vi "Autonomous Independent.vi"() -> ()   [LabVIEW 2012]
doc: "This VI is called when autonomous begins, and will automatically be terminated when autonomous ends. You can carry out timed or sensor driven robot movement independently without needing to return to the caller."
uses:
  <vilib>/Rock Robotics/WPI/Solenoid/WPI_SolenoidValue.ctl
  Robot Global Data.vi
  <vilib>/Rock Robotics/WPI/Joystick/WPI_JoystickGetSetRefNum.vi
  <vilib>/Rock Robotics/WPI/Solenoid/WPI_SolenoidSetEnum.vi
  <vilib>/addons/control/pid/pid.llb/PID (DBL).vi
  <vilib>/addons/control/pid/NI_PID_pid.lvlib
panel:
  in  "StraightPID gains 2":T1={"proportional gain (Kc)"=0.2, "integral time (Ti, min)"=0.0, "derivative time (Td, min)"=0.0} {"derivative time (Td, min)" format="%.3f"; "integral time (Ti, min)" format="%.3f"; "proportional gain (Kc)" format="%.3f"}
  in  "distance to bridge":dbl=4.1
  in  "Min Speed Bridge":dbl=0.1
  out "Distance Shoot":dbl[](array[numeric])=[0.5463065049614113, 0.4884233737596472] format="%#_4f"
  out "Distance Bridge":dbl[](array[numeric])=[15.640573318632855, 16.066427783902977] format="%#_4f"
  in  "Bridge approach\nSpeed":dbl=0.25
  in  "StraightPID gains":T1={"proportional gain (Kc)"=0.2, "integral time (Ti, min)"=0.0, "derivative time (Td, min)"=0.0} {"derivative time (Td, min)" format="%.3f"; "integral time (Ti, min)" format="%.3f"; "proportional gain (Kc)" format="%.3f"}
  in  "Shooter approach\nSpeed":dbl=-0.25
  out "Header":dbl
  in  "Min Speed Shoot":dbl=-0.1
  in  "Enum":enum16{"Straight", "Right", "Left", "Vision"}(ring)
  in  "PID gains":T1={"proportional gain (Kc)"=0.1, "integral time (Ti, min)"=0.0, "derivative time (Td, min)"=0.0} {"derivative time (Td, min)" format="%.3f"; "integral time (Ti, min)" format="%.3f"; "proportional gain (Kc)" format="%.3f"}
  out "Heading":dbl
  in  "Min Distance (ft)":dbl=3.25
  in  "inRange Power":dbl=-0.3
  out "Distance (ft)":dbl
  in  "inRange distance (ft)":dbl=4.0
  in  "Reverse Power":dbl=0.2
  in  "Camera Position":T2={"Radius (in)"=0.0, "Height (in)"=39.0, "Vertical Angle"=0.0}
  # "This assumes that the camera\nis facing directly out from the \ncenter of the robot"
  # "Distance from camera to \naxis of rotation on the robot"
  # "Example:"
  # "-0.1"
  # "4"
  # "0.1"
  # "-.25"
  # ".200"
  # ".25"
  # "Axis of rotation"
  # "Camera"
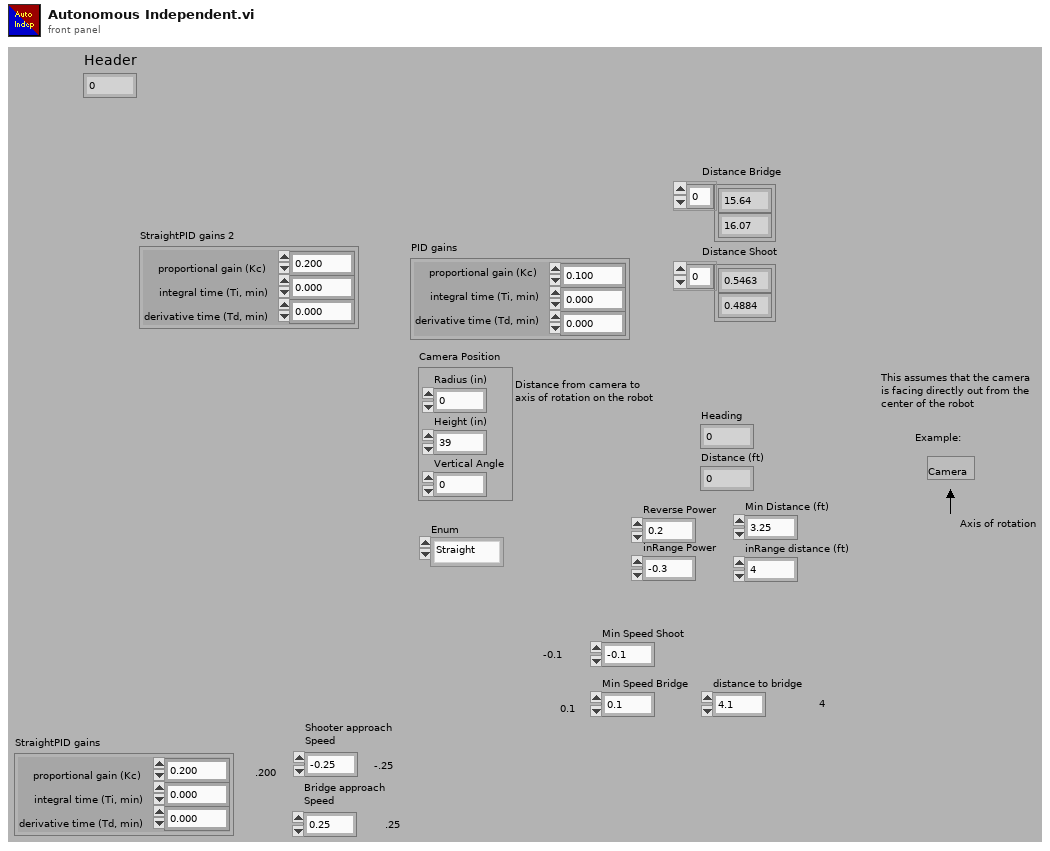
[diagram p1: front panel]
types:
  T1 = cluster{"proportional gain (Kc)":dbl, "integral time (Ti, min)":dbl, "derivative time (Td, min)":dbl}
  T2 = cluster{"Radius (in)":dbl, "Height (in)":dbl, "Vertical Angle":dbl}
  T3 = typedef "WPI_JoystickDevRef.ctl" = cluster{"Device":T4}
  T4 = typedef "WPI_JoystickDeviceEnum.ctl" = enum16{"USB 1", "USB 2", "USB 3", "USB 4", "Kinect 1", "Kinect 2"}
  T5 = cluster{"axis 1 (x)":dbl, "axis 2 (y)":dbl, "axis 3 (throttle)":dbl, "axis 4":dbl, "axis 5":dbl, "axis 6":dbl}
  T6 = typedef "WPI_MotorControlDeviceRef.ctl" = cluster{"DeviceStatus":errorcluster, "Type":enum16{"PWM", "CAN"}, "PWM":cluster{"Digital Module":T7, "PWM Channel":T8, "DeadBand":T9}, "CAN":cluster{"Device Number":u8, "Control Mode":T10, "Semaphore":T11, "Max Vout":dbl}, "Invert":bool, "TransformRef":T12, "InvTransformRef":T12}
  T7 = typedef "FPGA_TypedefDigitalModule.ctl" = enum16{"Digital Module 1", "Digital Module 2"}
  T8 = typedef "FPGA_DIOPWMChannel.ctl" = enum8{"PWM 1", "PWM 2", "PWM 3", "PWM 4", "PWM 5", "PWM 6", "PWM 7", "PWM 8", "PWM 9", "PWM 10", "Invalid"}
  T9 = typedef "WPI_PWMDeadband.ctl" = cluster{"Name":string, "maxPositivePwm":i32, "minPositivePwm":i32, "centerPwm":i32, "maxNegativePwm":i32, "minNegativePwm":i32, "angularRange":u16}
  T10 = typedef "WPI_CANJaguar_ControlMode.ctl" = enum8{"Percent VBus", "Current", "Speed", "Position", "Voltage"}
  T11 = typedef "Semaphore RefNum" = refnum<k1>
  T12 = typedef "WPI_PWMTransform_ConPane.ctl" = refnum<vi>
  T13 = typedef "WPI_SolenoidValue.ctl" = enum16{"Off", "On", "Forward", "Reverse"}
  T14 = typedef "WPI_SolenoidDevRef.ctl" = cluster{"DevStatus":errorcluster, "Solenoid Module":T15, "Forward Solenoid Channel":T16, "Reverse Solenoid Channel":T16}
  T15 = typedef "FPGA_TypedefSolenoidModule.ctl" = enum16{"Solenoid Module 1", "Solenoid Module 2"}
  T16 = typedef "WPI_SolenoidChannel.ctl" = enum8{"Solenoid 1", "Solenoid 2", "Solenoid 3", "Solenoid 4", "Solenoid 5", "Solenoid 6", "Solenoid 7", "Solenoid 8", "Invalid"}
  T17 = cluster{"Position":cluster{"X":dbl, "Y":dbl}, "Distance (ft)":dbl, "Angle Offset":dbl, "Bounding Box":cluster{"Left":dbl, "Top":dbl, "Right":dbl, "Bottom":dbl}}[]
  T18 = cluster{"Position":cluster{"X":dbl, "Y":dbl}, "Distance (ft)":dbl, "Angle Offset":dbl, "Bounding Box":cluster{"Left":dbl, "Top":dbl, "Right":dbl, "Bottom":dbl}}
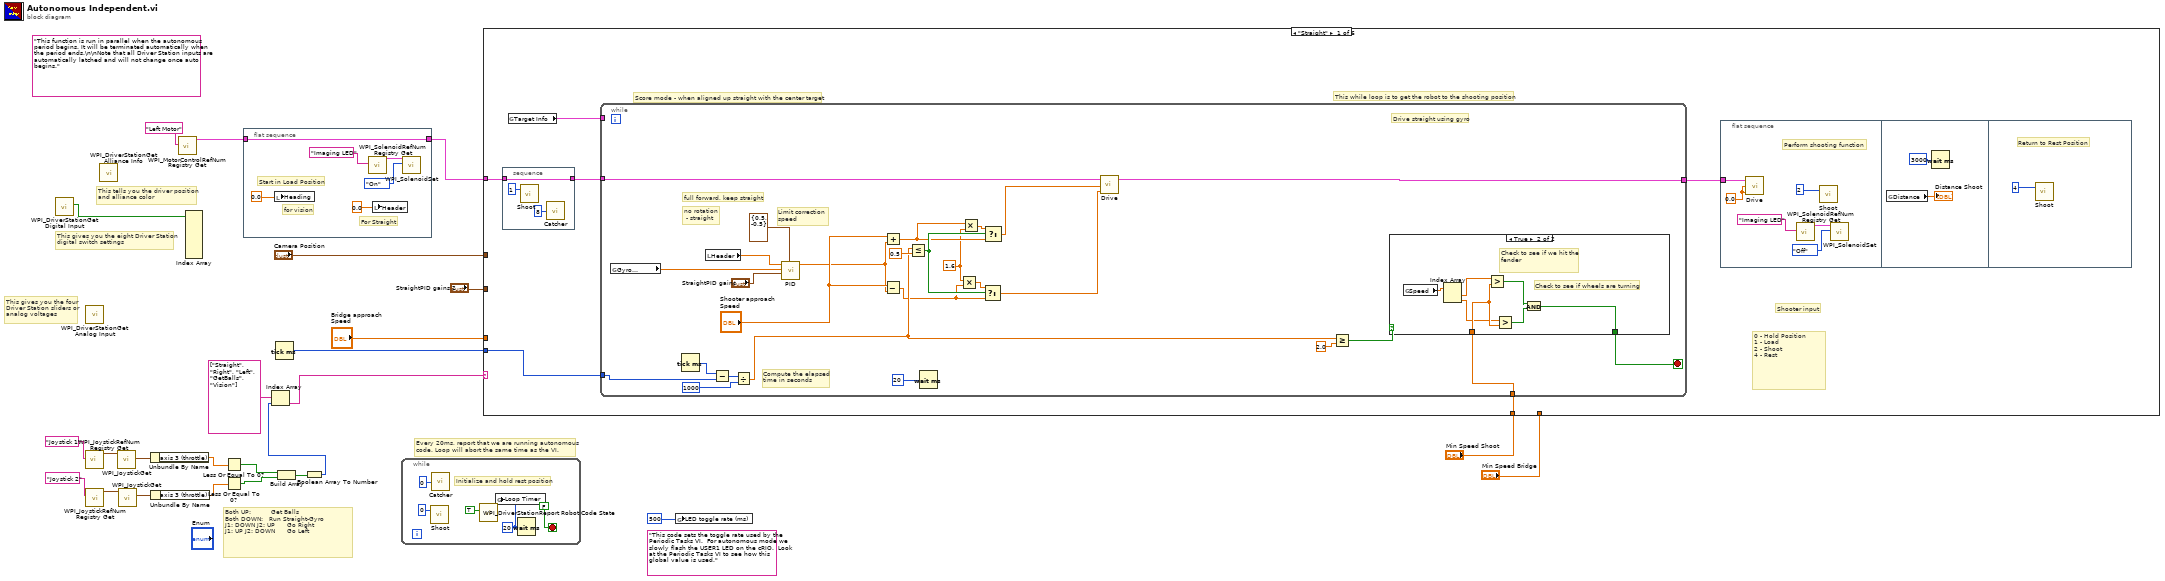
[diagram p0: block diagram]
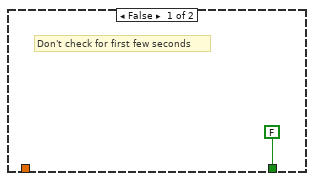
[diagram p2: hidden frame]
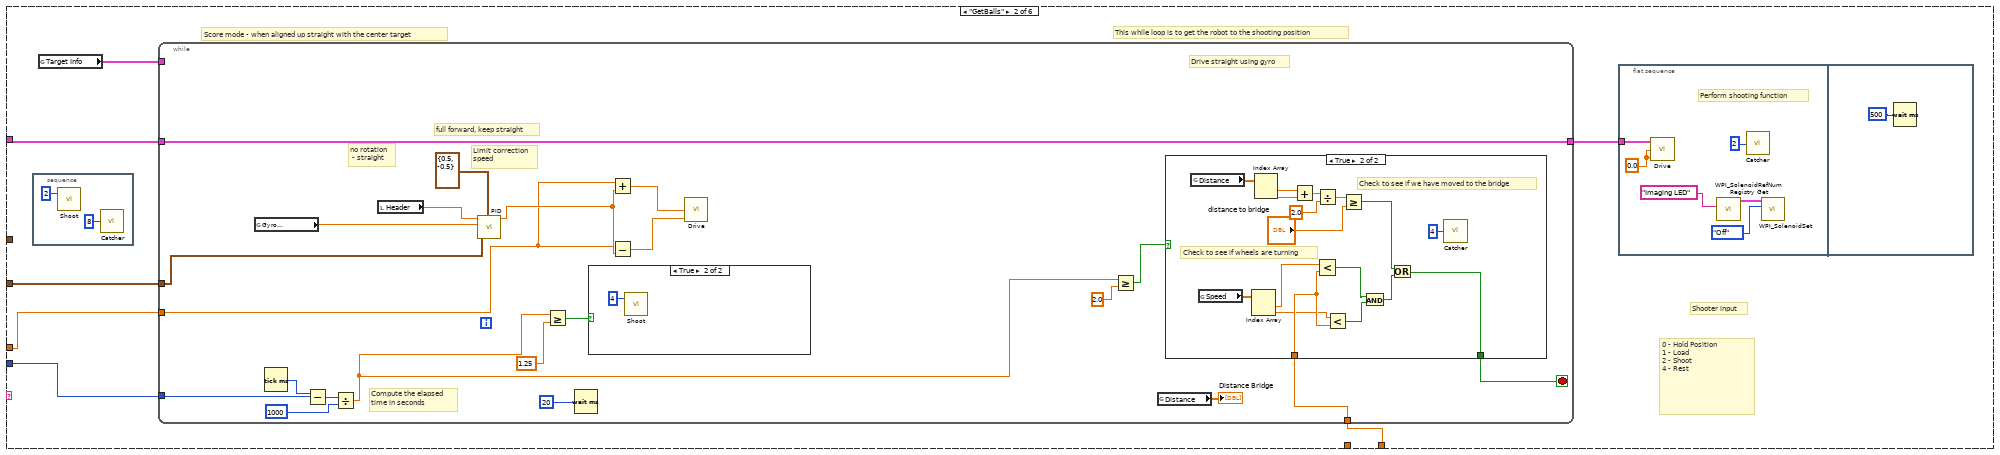
[diagram p3: hidden frame]
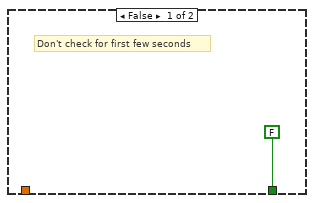
[diagram p5: hidden frame]
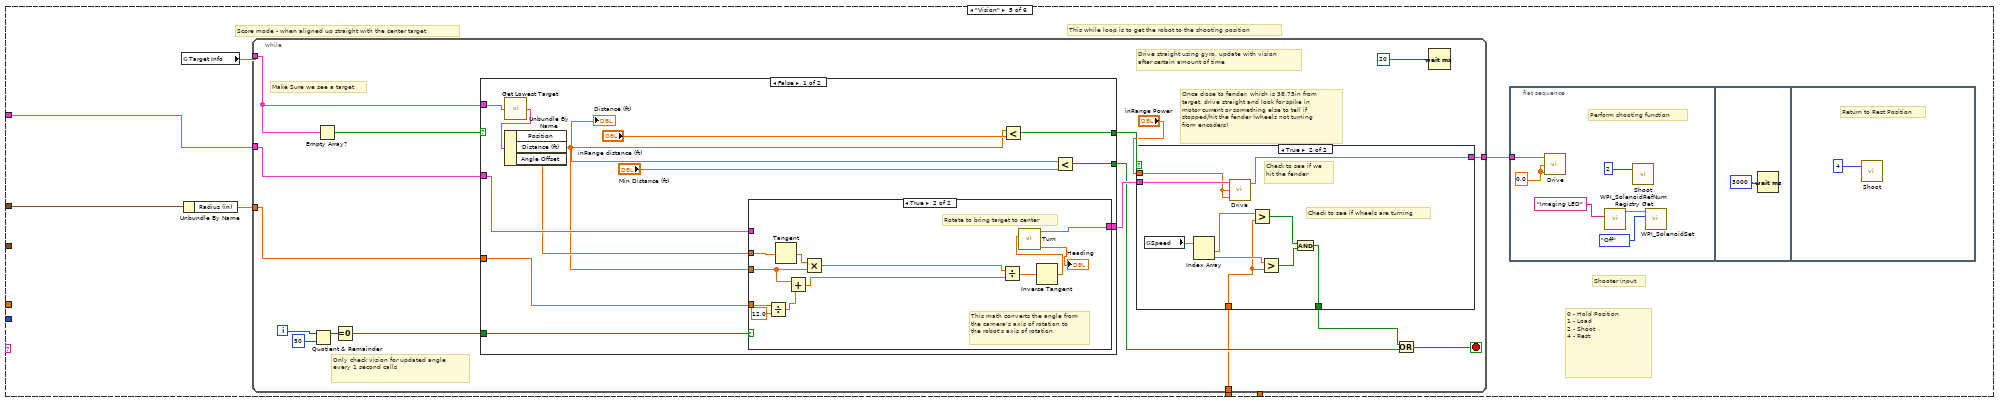
[diagram p8: hidden frame]
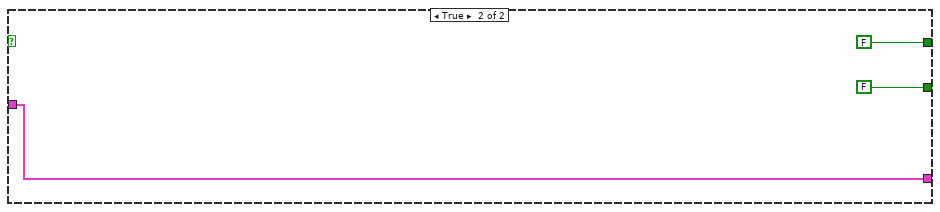
[diagram p10: hidden frame]
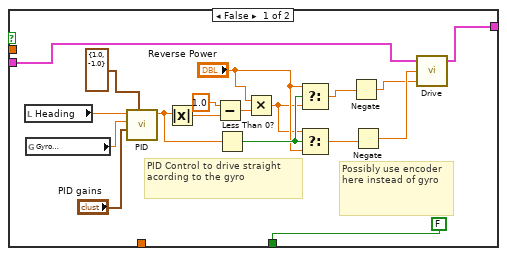
[diagram p11: hidden frame]
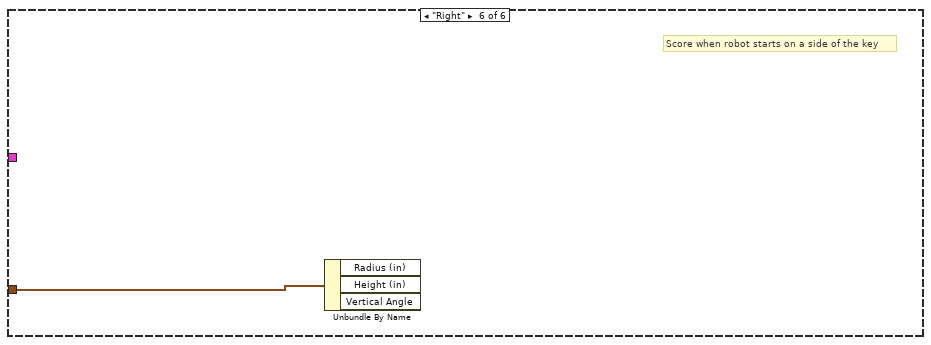
[diagram p12: hidden frame]
diagram:
  (unwired) "This code sets the toggle rate used by the Periodic Tasks VI.  For autonomous mode we slowly flash the USER1 LED on the cRIO.  Look at the Periodic Tasks VI to see how this global value is used."
  (unwired) "This function is run in parallel when the autonomous period begins. It will be terminated automatically when the period ends.\n\nNote that all Driver Station inputs are automatically latched and will not change once auto begins."
  # "Both UP:          Get Balls\nBoth DOWN:   Run Straight-Gyro\nJ1: DOWN J2: UP      Go Right\nJ1: UP J2: DOWN      Go Left"
  # "Every 20ms, report that we are running autonomous\ncode. Loop will abort the same time as the VI."
  # "This tells you the driver position\nand alliance color"
  # "This gives you the eight Driver Station\ndigital switch settings"
  # "This gives you the four\nDriver Station sliders or\nanalog voltages"
  n1 = call <vilib>:"WPI_DriverStationGet Digital Input.vi"() -> ("Driver Station Digital Input (1-8)"=w25:bool[])  [unwired: 11 out]
  n2 = call <vilib>:"WPI_JoystickRefNum Registry Get.vi"("refnum name"="Joystick 1") -> ("JoystickDevRef"=w14:T3)  [unwired: 1 in, 9 out]
  n3 = call <vilib>:"WPI_DriverStationGet Analog Input.vi"() -> ()  [unwired: 12 out]
  n4 = call <vilib>:"WPI_JoystickRefNum Registry Get.vi"("refnum name"="Joystick 2") -> ("JoystickDevRef"=w11:T3)  [unwired: 1 in, 9 out]
  n5 = call <vilib>:"WPI_DriverStationGet Alliance Info.vi"() -> ()  [unwired: 12 out]
  n6 = call <vilib>:"WPI_JoystickGet.vi"("JoystickDevRef"=w14) -> ("Axes"=w15:T5)  [unwired: 1 in, 5 out]
  n7 = call <vilib>:"WPI_JoystickGet.vi"("JoystickDevRef"=w11) -> ("Axes"=w10:T5)  [unwired: 1 in, 5 out]
  n8 = Unbundle By Name(w15) -> ("axis 3 (throttle)"=w13:dbl)
  n9 = Unbundle By Name(w10) -> ("axis 3 (throttle)"=w12:dbl)
  n10 = call <vilib>:"WPI_MotorControlRefNum Registry Get.vi"("refnum name"="Left Motor") -> ("MotorControlDevRef"=w5:T6)  [unwired: 9 in, 1 out]
  n11 = Index Array(array=w25) -> ()  [unwired: 8 in, 8 out]
  n12 = Less Or Equal To 0?(x=w13) -> (x <= 0?=w6:bool)
  n13 = Less Or Equal To 0?(x=w12) -> (x <= 0?=w7:bool)
  n14 = flat-sequence {
    tunnel: [w31] -> w4
    tunnel: w5 -> [w31]
    frame #0 {
      # "For Straight"
      # "for vision"
      # "Start in Load Position"
      n15 = local write "Heading"(0.0 ("Heading")) -> ()
      n16 = call <vilib>:"WPI_SolenoidRefNum Registry Get.vi"("refnum name"="Imaging LED") -> ("SolenoidDevRef"=w29:T14)  [unwired: 9 in, 1 out]
      n17 = local write "Header"(0.0 ("Header")) -> ()
      n18 = call-poly <vilib>:"WPI_SolenoidSet.vi"("Value"=WPI_SolenoidValue."On", "SolenoidDevRef"=w29) -> ()  [unwired: 8 in, 2 out]
    }
  }
  n19 = Tick Count (ms)() -> (millisecond timer value=w18:u32)
  n20 = Build Array(w6, w7) -> (w8:bool[])
  n21 = Boolean Array To Number(Boolean array=w8) -> (number=w22:u32)
  n22 = Index Array(array=string[] ["Straight", "Right", "Left", "GetBalls", "Vision"], index=w22) -> (element=w21:string)
  n23 = while {
    stop <- FALSE stop-if-true
    w33 = u32 20 ("milliseconds to wait")
    # "Initialize and hold rest position"
    n24 = call "Shoot.vi"("Shooter Position (0 to 8)"=i8 0 ("Shooter Position (0 to 4)")) -> ()  [unwired: 1 in, 2 out]
    n25 = call "Catcher.vi"("Catcher Position"=i8 0) -> ()
    n26 = call <vilib>:"WPI_DriverStationReport Robot Code State.vi"("Autonomous"=TRUE) -> ()  [unwired: 10 in, 1 out]
    n27 = global write "Robot Global Data.vi" "Loop Timer"(w33) -> ()
    n28 = Wait (ms)(milliseconds to wait=w33) -> ()  [unwired: 1 out]
  }
  n29 = case shown="\"Straight\"" w21 {
    tunnel: w4 -> [w38 w94 _ _ w151 _]
    tunnel: "Camera Position" -> [_ _ _ _ w150 w234]
    tunnel: w18 -> [w40 w93 _ _ _ _]
    tunnel: "Min Speed Shoot" -> [w39 _ _ _ w147 _]
    tunnel: "Bridge approach\nSpeed" -> [_ w92 _ _ _ _]
    tunnel: "Min Speed Bridge" -> [_ w91 _ _ _ _]
    tunnel: "StraightPID gains 2" -> [_ w90 _ _ _ _]
    frame "Straight" {
      # "Shooter input"
      # "0 - Hold Position\n1 - Load\n2 - Shoot\n4 - Rest"
      # "This while loop is to get the robot to the shooting position"
      # "Score mode - when aligned up straight with the center target"
      n30 = stacked-sequence {
        tunnel: [w43] -> w37
        tunnel: w38 -> [w43]
        frame #0 {
          n31 = call "Shoot.vi"("Shooter Position (0 to 8)"=i8 1 ("Shooter Position (0 to 4)")) -> ()  [unwired: 1 in, 2 out]
          n32 = call "Catcher.vi"("Catcher Position"=i8 8) -> ()
        }
      }
      n33 = global read "Robot Global Data.vi" "Target Info"() -> (w42:T17)
      n34 = while {
        tunnel: w42 -> [_]
        tunnel: w37 -> [w70]
        tunnel: [w69] -> w41
        tunnel: w40 -> [w77]
        tunnel: w39 -> [w76]
        stop <- w75 stop-if-true
        w56 = 1.6 ("y")
        # "full forward, keep straight"
        # "Limit correction\nspeed"
        # "no rotation\n - straight"
        # "Compute the elapsed\ntime in seconds"
        # "Drive straight using gyro"
        n35 = global read "Robot Global Data.vi" "Gyro\nAngle"() -> (w67:dbl)
        n36 = Tick Count (ms)() -> (millisecond timer value=w80:u32)
        n37 = local read "Header"() -> (w65:dbl)
        n38 = Subtract(x=w80, y=w77) -> (x-y=w78:u32)
        n39 = Divide(x=w78, y=u32 1000 ("milliseconds to wait")) -> (x/y=w71:dbl)
        n40 = call-poly <vilib>:"PID.vi"("output range"=cluster{"output high":dbl, "output low":dbl} {"output high"=0.5, "output low"=-0.5}, "PID gains"="StraightPID gains", "process variable"=w67, "setpoint"=w65) -> ("output"=w62:dbl)  [unwired: 2 in, 5 out]
        n41 = Subtract(x="Shooter approach\nSpeed", y=w62) -> (x-y=w55:dbl)
        n42 = Add(x="Shooter approach\nSpeed", y=w62) -> (x+y=w58:dbl)
        n43 = Less Or Equal?(x=w71, y=0.5) -> (x <= y?=w63:bool)
        n44 = Wait (ms)(milliseconds to wait=u32 20) -> ()  [unwired: 1 out]
        n45 = Multiply(x=w56, y=w55) -> (x*y=w57:dbl)
        n46 = Multiply(x=w58, y=w56) -> (x*y=w59:dbl)
        n47 = Select(t=w57, s=w63, f=w55) -> (s? t:f=w60:dbl)
        n48 = Select(t=w59, s=w63, f=w58) -> (s? t:f=w61:dbl)
        n49 = call "Drive.vi"("Right Motor IN"=w60, "Left Motor IN"=w61, "Motor DevRef"=w70) -> ("Motor DevRef"=w69:T6)  [unwired: 2 in]
        n50 = Greater Or Equal?(x=w71, y=2.0) -> (x >= y?=w74:bool)
        n51 = case shown="True" w74 {
          tunnel: w76 -> [_ w89]
          tunnel: [FALSE w88] -> w75
          frame False {
            # "Don't check for first few seconds"
          }
          frame True {
            # "Check to see if wheels are turning"
            # "Check to see if we hit the fender"
            n52 = global read "Robot Global Data.vi" "Speed"() -> (w85:dbl[])
            n53 = Index Array(array=w85) -> (element #1=w84:dbl, element #2=w83:dbl)  [unwired: 2 in]
            n54 = Greater?(x=w84, y=w89) -> (0:w87:bool)
            n55 = Greater?(x=w83, y=w89) -> (0:w86:bool)
            n56 = And(x=w87, y=w86) -> (x .and. y?=w88:bool)
          }
        }
      }
      n57 = flat-sequence {
        tunnel: w41 -> [w50]
        frame #0 {
          w51 = 0.0 ("RightSpeed")
          # "Perform shooting function"
          n58 = call "Drive.vi"("Right Motor IN"=w51, "Left Motor IN"=w51, "Motor DevRef"=w50) -> ()  [unwired: 2 in, 1 out]
          n59 = call <vilib>:"WPI_SolenoidRefNum Registry Get.vi"("refnum name"="Imaging LED") -> ("SolenoidDevRef"=w48:T14)  [unwired: 9 in, 1 out]
          n60 = call "Shoot.vi"("Shooter Position (0 to 8)"=i8 2 ("Shooter Position (0 to 3)")) -> ()  [unwired: 1 in, 2 out]
          n61 = call-poly <vilib>:"WPI_SolenoidSet.vi"("Value"=WPI_SolenoidValue."Off", "SolenoidDevRef"=w48) -> ()  [unwired: 8 in, 2 out]
        }
        frame #1 {
          n62 = global read "Robot Global Data.vi" "Distance"() -> (→"Distance Shoot":dbl[])
          n63 = Wait (ms)(milliseconds to wait=u32 3000) -> ()  [unwired: 1 out]
        }
        frame #2 {
          # "Return to Rest Position"
          n64 = call "Shoot.vi"("Shooter Position (0 to 8)"=i8 4 ("Shooter Position (0 to 3)")) -> ()  [unwired: 1 in, 2 out]
        }
      }
    }
    frame "GetBalls" {
      # "Shooter input"
      # "0 - Hold Position\n1 - Load\n2 - Shoot\n4 - Rest"
      # "This while loop is to get the robot to the shooting position"
      # "Score mode - when aligned up straight with the center target"
      n65 = stacked-sequence {
        frame #0 {
          n66 = call "Shoot.vi"("Shooter Position (0 to 8)"=i8 2 ("Shooter Position (0 to 4)")) -> ()  [unwired: 1 in, 2 out]
          n67 = call "Catcher.vi"("Catcher Position"=i8 8) -> ()
        }
      }
      n68 = global read "Robot Global Data.vi" "Target Info"() -> (w96:T17)
      n69 = while {
        tunnel: w96 -> [_]
        tunnel: w94 -> [w121]
        tunnel: [w121] -> w95
        tunnel: w93 -> [w123]
        tunnel: w91 -> [w122]
        tunnel: w92 -> [w111]
        tunnel: w90 -> [w110]
        stop <- w120 stop-if-true
        # "Limit correction\nspeed"
        # "no rotation\n - straight"
        # "full forward, keep straight"
        # "Compute the elapsed\ntime in seconds"
        # "Drive straight using gyro"
        n70 = global read "Robot Global Data.vi" "Gyro\nAngle"() -> (w119:dbl)
        n71 = Tick Count (ms)() -> (millisecond timer value=w126:u32)
        n72 = Subtract(x=w126, y=w123) -> (x-y=w124:u32)
        n73 = Divide(x=w124, y=u32 1000 ("milliseconds to wait")) -> (x/y=w107:dbl)
        n74 = local read "Header"() -> (w117:dbl)
        n75 = call-poly <vilib>:"PID.vi"("output range"=cluster{"output high":dbl, "output low":dbl} {"output high"=0.5, "output low"=-0.5}, "PID gains"=w110, "process variable"=w119, "setpoint"=w117) -> ("output"=w116:dbl)  [unwired: 2 in, 5 out]
        n76 = Greater Or Equal?(x=w107, y=1.25) -> (x >= y?=w106:bool)
        n77 = Wait (ms)(milliseconds to wait=u32 20) -> ()  [unwired: 1 out]
        n78 = case shown="True" w106 {
          frame False {
          }
          frame True {
            n79 = call "Shoot.vi"("Shooter Position (0 to 8)"=i8 4 ("Shooter Position (0 to 4)")) -> ()  [unwired: 1 in, 2 out]
          }
        }
        n80 = Subtract(x=w111, y=w116) -> (x-y=w114:dbl)
        n81 = Add(x=w111, y=w116) -> (x+y=w115:dbl)
        n82 = call "Drive.vi"("Right Motor IN"=w114, "Left Motor IN"=w115) -> ()  [unwired: 3 in, 1 out]
        n83 = Greater Or Equal?(x=w107, y=2.0) -> (x >= y?=w113:bool)
        n84 = global read "Robot Global Data.vi" "Distance"() -> (→"Distance Bridge":dbl[])
        n85 = case shown="True" w113 {
          tunnel: w122 -> [_ w146]
          tunnel: [FALSE w131] -> w120
          frame False {
            # "Don't check for first few seconds"
          }
          frame True {
            # "Check to see if we have moved to the bridge"
            # "Check to see if wheels are turning"
            n86 = global read "Robot Global Data.vi" "Distance"() -> (w140:dbl[])
            n87 = global read "Robot Global Data.vi" "Speed"() -> (w143:dbl[])
            n88 = Index Array(array=w143) -> (element #1=w142:dbl, element #2=w141:dbl)  [unwired: 2 in]
            n89 = Index Array(array=w140) -> (element #1=w139:dbl, element #2=w138:dbl)  [unwired: 2 in]
            n90 = Add(x=w139, y=w138) -> (x+y=w137:dbl)
            n91 = Less?(x=w142, y=w146) -> (x < y?=w145:bool)
            n92 = Divide(x=w137, y=2.0) -> (x/y=w135:dbl)
            n93 = Less?(x=w141, y=w146) -> (x < y?=w144:bool)
            n94 = Greater Or Equal?(x=w135, y="distance to bridge") -> (x >= y?=w132:bool)
            n95 = And(x=w145, y=w144) -> (x .and. y?=w133:bool)
            n96 = Or(x=w132, y=w133) -> (x .or. y?=w131:bool)
            n97 = call "Catcher.vi"("Catcher Position"=i8 4) -> ()
          }
        }
      }
      n98 = flat-sequence {
        tunnel: w95 -> [w103]
        frame #0 {
          w104 = 0.0 ("RightSpeed")
          # "Perform shooting function"
          n99 = call "Drive.vi"("Right Motor IN"=w104, "Left Motor IN"=w104, "Motor DevRef"=w103) -> ()  [unwired: 2 in, 1 out]
          n100 = call <vilib>:"WPI_SolenoidRefNum Registry Get.vi"("refnum name"="Imaging LED") -> ("SolenoidDevRef"=w102:T14)  [unwired: 9 in, 1 out]
          n101 = call "Catcher.vi"("Catcher Position"=i8 2) -> ()
          n102 = call-poly <vilib>:"WPI_SolenoidSet.vi"("Value"=WPI_SolenoidValue."Off", "SolenoidDevRef"=w102) -> ()  [unwired: 8 in, 2 out]
        }
        frame #1 {
          n103 = Wait (ms)(milliseconds to wait=u32 500) -> ()  [unwired: 1 out]
        }
      }
    }
    frame Default {
      # "Default, Do nothing"
    }
    frame "Left" {
    }
    frame "Vision" {
      # "Shooter input"
      # "0 - Hold Position\n1 - Load\n2 - Shoot\n4 - Rest"
      # "This while loop is to get the robot to the shooting position"
      # "Score mode - when aligned up straight with the center target"
      n104 = global read "Robot Global Data.vi" "Target Info"() -> (w152:T17)
      n105 = Unbundle By Name(w150) -> ("Radius (in)"=w149:dbl)
      n106 = while {
        tunnel: w152 -> [w168]
        tunnel: w151 -> [w175]
        tunnel: w149 -> [w169]
        tunnel: [w163] -> w148
        tunnel: w147 -> [w161]
        i -> [w177]
        stop <- w166 stop-if-true
        # "Only check vision for updated angle every 1 second calls"
        # "Make Sure we see a target"
        # "Once close to fender, which is 38.75in from target, drive straight and look for spike in motor current or something else to tell if stopped/hit the fender (wheels not turning from encoders)"
        # "Drive straight using gyro, update with vision \nafter certain amount of time"
        n107 = Quotient & Remainder(x=w177, y=50) -> (x-y*floor(x/y)=w176:i32)  [unwired: 1 out]
        n108 = Empty Array?(array=w168) -> (empty?=w167:bool)
        n109 = Equal To 0?(x=w176) -> (x = 0?=w170:bool)
        n110 = case shown="False" w167 {
          tunnel: w175 -> [w189 w203]
          tunnel: [w187 w203] -> w174
          tunnel: [w185 FALSE] -> w173
          tunnel: [w183 FALSE] -> w165
          tunnel: w168 -> [w178 _]
          tunnel: w170 -> [w182 _]
          tunnel: w169 -> [w181 _]
          frame False {
            n111 = call "Get Lowest Target.vi"("Target Info"=w178) -> ("Lowest Target Info"=w179:T18)
            n112 = Unbundle By Name(w179) -> ("Distance (ft)"=w180:dbl, "Angle Offset"=w188:dbl)  [unwired: 1 out]
            "Distance (ft)" <- w180
            n113 = case shown="True" w182 {
              tunnel: w189 -> [w190 _]
              tunnel: w188 -> [_ w202]
              tunnel: [w190 w193] -> w187
              tunnel: w181 -> [_ w196]
              tunnel: w180 -> [_ w199]
              frame False {
              }
              frame True {
                # "This math converts the angle from the camera's axis of rotation to the robot's axis of rotation"
                # "Rotate to bring target to center"
                n114 = Divide(x=w196, y=12.0) -> (x/y=w195:dbl)
                n115 = Tangent(1:w202) -> (0:w201:dbl)
                n116 = Add(x=w199, y=w195) -> (x+y=w198:dbl)
                n117 = Multiply(x=w201, y=w199) -> (x*y=w200:dbl)
                n118 = Divide(x=w200, y=w198) -> (x/y=w197:dbl)
                n119 = Inverse Tangent(1:w197) -> (0:w192:dbl)
                n120 = call "Turn.vi"("Heading Change (Degrees)"=w192) -> ("Actual Heading (Degrees)"=→"Heading":dbl, "Motor DevRef"=w193:T6)  [unwired: 9 in]
              }
            }
            n121 = Less?(x=w180, y="inRange distance (ft)") -> (x < y?=w185:bool)
            n122 = Less?(x=w180, y="Min Distance (ft)") -> (x < y?=w183:bool)
          }
          frame True {
          }
        }
        n123 = case shown="True" w173 {
          tunnel: w174 -> [w206 w229]
          tunnel: [FALSE w231] -> w164
          tunnel: [w207 w230] -> w163
          tunnel: "inRange Power" -> [_ w225]
          tunnel: w161 -> [_ w224]
          frame False {
            # "Possibly use encoder here instead of gyro"
            # "PID Control to drive straight acording to the gyro"
            n124 = local read "Heading"() -> (w223:dbl)
            n125 = global read "Robot Global Data.vi" "Gyro\nAngle"() -> (w209:dbl)
            n126 = call-poly <vilib>:"PID.vi"("output range"=cluster{"output high":dbl, "output low":dbl} {"output high"=1.0, "output low"=-1.0}, "PID gains"="PID gains", "process variable"=w209, "setpoint"=w223) -> ("output"=w219:dbl)  [unwired: 6 in, 1 out]
            n127 = Absolute Value(x=w219) -> (abs(x)=w217:dbl)
            n128 = Subtract(x=1.0, y=w217) -> (x-y=w216:dbl)
            n129 = Less Than 0?(x=w219) -> (x < 0?=w220:bool)
            n130 = Multiply(x="Reverse Power", y=w216) -> (x*y=w214:dbl)
            n131 = Select(t="Reverse Power", s=w220, f=w214) -> (s? t:f=w211:dbl)
            n132 = Select(t=w214, s=w220, f="Reverse Power") -> (s? t:f=w213:dbl)
            n133 = Negate(x=w211) -> (-x=w210:dbl)
            n134 = Negate(x=w213) -> (-x=w212:dbl)
            n135 = call "Drive.vi"("Right Motor IN"=w210, "Left Motor IN"=w212, "Motor DevRef"=w206) -> ("Motor DevRef"=w207:T6)  [unwired: 2 in]
          }
          frame True {
            # "Check to see if wheels are turning"
            # "Check to see if we hit the fender"
            n136 = global read "Robot Global Data.vi" "Speed"() -> (w228:dbl[])
            n137 = Index Array(array=w228) -> (element #1=w227:dbl, element #2=w226:dbl)  [unwired: 2 in]
            n138 = call "Drive.vi"("Right Motor IN"=w225, "Left Motor IN"=w225, "Motor DevRef"=w229) -> ("Motor DevRef"=w230:T6)  [unwired: 2 in]
            n139 = Greater?(x=w227, y=w224) -> (0:w233:bool)
            n140 = Greater?(x=w226, y=w224) -> (0:w232:bool)
            n141 = And(x=w233, y=w232) -> (x .and. y?=w231:bool)
          }
        }
        n142 = Or(x=w164, y=w165) -> (x .or. y?=w166:bool)
        n143 = Wait (ms)(milliseconds to wait=u32 20) -> ()  [unwired: 1 out]
      }
      n144 = flat-sequence {
        tunnel: w148 -> [w157]
        frame #0 {
          w158 = 0.0 ("RightSpeed")
          # "Perform shooting function"
          n145 = call "Drive.vi"("Right Motor IN"=w158, "Left Motor IN"=w158, "Motor DevRef"=w157) -> ()  [unwired: 2 in, 1 out]
          n146 = call <vilib>:"WPI_SolenoidRefNum Registry Get.vi"("refnum name"="Imaging LED") -> ("SolenoidDevRef"=w155:T14)  [unwired: 9 in, 1 out]
          n147 = call "Shoot.vi"("Shooter Position (0 to 8)"=i8 2 ("Shooter Position (0 to 3)")) -> ()  [unwired: 1 in, 2 out]
          n148 = call-poly <vilib>:"WPI_SolenoidSet.vi"("Value"=WPI_SolenoidValue."Off", "SolenoidDevRef"=w155) -> ()  [unwired: 8 in, 2 out]
        }
        frame #1 {
          n149 = Wait (ms)(milliseconds to wait=u32 3000) -> ()  [unwired: 1 out]
        }
        frame #2 {
          # "Return to Rest Position"
          n150 = call "Shoot.vi"("Shooter Position (0 to 8)"=i8 4 ("Shooter Position (0 to 3)")) -> ()  [unwired: 1 in, 2 out]
        }
      }
    }
    frame "Right" {
      # "Score when robot starts on a side of the key"
      n151 = Unbundle By Name(w234) -> ()  [unwired: 3 out]
    }
  }
  n152 = global write "Robot Global Data.vi" "LED toggle rate (ms)"(u32 500 ("LED ms toggle rate")) -> ()
